vi "HEWH Temp Decline FGV.vi"(8 "error in (no error)":errorcluster, 10 "Last Draw TC Tree AVG Decline Amount (Degrees F)":dbl, 11 "TC Tree (AVG)":dbl) -> (0 "error out":errorcluster, 3 "Temp Decline Complete":bool)   [LabVIEW 2016]
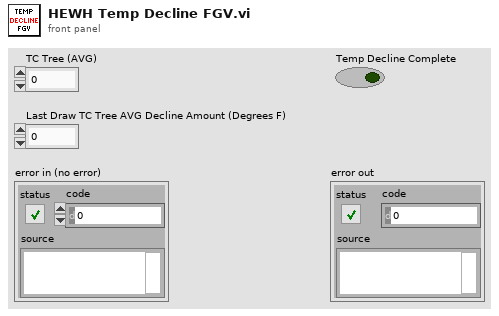
[diagram p1: front panel]
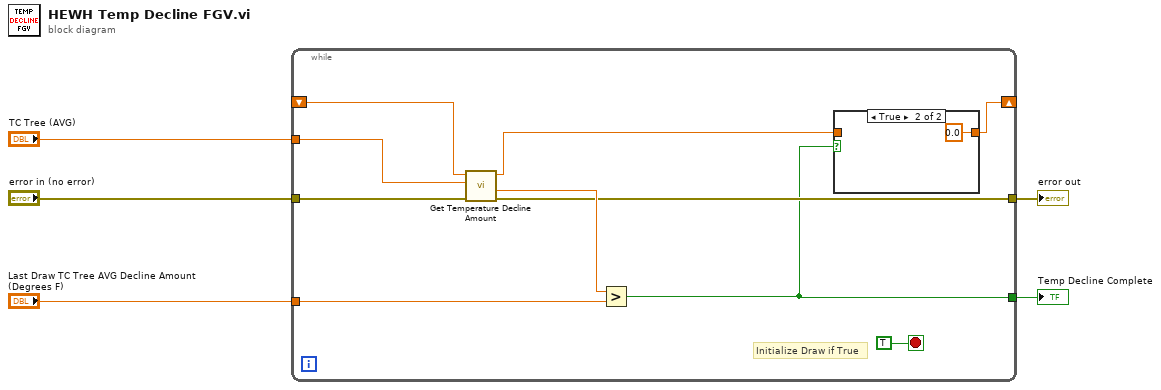
[diagram p0: block diagram]
diagram:
  n1 = while {
    tunnel: "error in (no error)" -> [w15]
    tunnel: "Last Draw TC Tree AVG Decline Amount (Degrees F)" -> [w13]
    tunnel: "TC Tree (AVG)" -> [w12]
    shift-right: [w7] -> _
    shift-left: _ -> [w11]
    tunnel: [w9] -> w4
    tunnel: [w6] -> w5
    stop <- TRUE stop-if-true
    # "Initialize Draw if True"
    n2 = call "Get Temperature Decline Amount.vi"("Error In"=w15, "TC Tree (AVG)"=w12, "Starting Temp Decline Input"=w11) -> ("Error Out"=w9:errorcluster, "Current Temp Decline Amout"=w14:dbl, "Starting Temp Decline Output"=w8:dbl)  [unwired: 5 in, 1 out]
    n3 = Greater?(x=w14, y=w13) -> (0:w6:bool)
    n4 = case shown="True" w6 {
      tunnel: w8 -> [w16 _]
      tunnel: [w16 0.0 ("Starting Temp Decline Output")] -> w7
      frame False {
      }
      frame True {
      }
    }
  }
  "Temp Decline Complete" <- w5
  "error out" <- w4
